vi "hReadChannels-UandP.vi"(0 "FPGA VI Reference In":refnum<k20>, 1 "SavGol side points":i32=10, 3 "Use Voltage or Power for AO?":bool, 4 "order polynomial":i32=2, 5 "Nsamples":u32=10000, 6 "error in":errorcluster, 8 "output cluster":T3, 9 "No. Of Samples to average":i32=5, 10 "variables cluster":T2, 11 "Calc Selection":u16(ring)=2 items=["0.4 ms", "0.8 ms", "1.6 ms", "3.2 ms", "6.4 ms", "12.8 ms"], 14 "skip feedback":bool) -> (2 "Fehler":bool, 13 "AdjustedArray":sgl[][](array[numeric]), 17 "loop DAQ timing":dbl, 18 "single channel voltage array":dbl[](array[numeric]), 19 "real time P_rad array":dbl[](array[numeric]), 20 "FPGA VI Reference Out":refnum<k20>, 22 "PowerArray":sgl[][](array[numeric]), 25 "RawArray":sgl[][](array[numeric]), 26 "error out":errorcluster)   [LabVIEW 2014]
doc: "startet das einlesen und führt dies bis n Samples aus\nHier mit FIFO und IRQ."
uses:
  <vilib>/Utility/error.llb/Error Cluster From Error Code.vi
  <vilib>/rvi/errors/niLvFpgaAdjustHostInterfaceError.vi
  <vilib>/RVI Host/nirviSupport.llb/nirviErrorClusterFromErrorCode.vi
  <vilib>/rvi/interface/nirviReadWriteControl/nirviReadWriteControl.xnode
  FPGA Bitfiles/W7XBolo2017_FPGATarget_fmain2014_DACRangeVoltage.lvbitx
  f_main_2014.vi
  <vilib>/rvi/interface/nirviMethod/nirviMethod.xnode
  NiFpgaLv.dll
  <vilib>/rvi/interface/nirviMethod/StockFPGA_InlinedMethodWaitForMultipleIRQ.vi
  <vilib>/FPGAPlugInAG/PCI-7813R/niLvFpga_WaitOnIrq_PCI-7813R.vi
  <vilib>/FPGAPlugInAG/PCI-7813R/niLvFpga_AcknowledgeIrq_PCI-7813R.vi
  <vilib>/FPGAPlugInAG/PCI-7813R/niLvFpga_ReadFifo_PCI-7813R.vi
  <vilib>/rvi/errors/niLvFpgaMergeErrorWithErrorCode.vi
panel:
  in  "Tab Control":T1(tab)
  out "16bit integer voltage sample":i16[](array[numeric])
  out "Timed Out":bool
  out "STOP?":bool
  out "Elements Remaining":u32
  out "single channel voltage":sgl
  out "single channel voltage * factor":dbl
  out "empty sample array":dbl[](array[numeric])
  out "Nsamples array":i64[](array[numeric])
  out "new level of override":i32=1565
  out "last U sample":sgl[](array[numeric])=[-7.323455e-08, 6.4667313e-07, 1.2200326e-06, -9.891577e-07, -1.4648394e-06, 8.4836154e-07, 0.0, -1.0253722e-06, -6.349012e-07, 2.9421412e-06, 1.8309802e-06, -1.6723759e-06, -8.0589206e-07, 1.2935698e-06, 1.2819655e-06, -1.355093e-06, -3.7858263e-07, 5.865097e-07, 5.370006e-07, -3.6600977e-07, 0.0, -4.235832e-06, 7.87382e-07, -8.300087e-07, -2.3216009e-07, 6.100163e-07, 4.6361237e-07, -4.2733737e-07, -1.1170097e-06, 4.6361237e-07, 6.4709224e-07, -9.032898e-07, 0.0, -3.600493e-07, -9.394251e-07, 7.939525e-07, 9.028241e-07, -9.2692676e-07, 6.595068e-07, -1.5255064e-06, -1.1291402e-06, 1.257381e-06, -1.1108303e-06, 1.4649238e-06, -8.564442e-08, -5.254149e-07, 5.859509e-07, -5.5879357e-10, -5.3096096e-07, 1.4771707e-06, 1.0997057e-07, -1.416197e-06, -6.2856355e-07, -8.4228816e-07, -1.6051717e-06, -8.0560335e-07, -2.3067928e-06, -1.1781231e-06, 1.4042482e-06, -1.1242553e-05, -2.111881e-06, 1.9225524e-06, -6.4575115e-06, 2.1361745e-07, 2.5024683e-06, -3.6619604e-06, -2.1238252e-06, -3.6375504e-06, -2.7460046e-06, 1.2200326e-06, 1.1045952e-06, -8.5447914e-07, -2.282681e-06, 0.0, 2.4409965e-06, 6.100163e-07, -5.0041825e-07, -1.842957e-06, -3.2471494e-06, -8.7925235e-07, 1.5277057e-05, 3.460478e-06, 2.8060748e-07, -2.3826956e-07, -2.3319571e-06, 1.3062544e-06, 5.428121e-07, 0.0, 6.6523904e-07, -1.2820121e-07, -2.563931e-06, -7.8128653e-07, -1.5884638e-07, 2.1481887e-06, 3.747493e-06, 4.270114e-07, -1.0980293e-07, -7.0789827e-07, -2.3180618e-07, 4.3368087e-19, -1.2810342e-07, 4.8801303e-07, 6.8413095e-07, 3.054738e-07, 1.830794e-07, 4.0261074e-07, -1.3440848e-07, -6.469898e-07, -8.1180593e-07, 7.629387e-07, 9.583147e-07, -1.2207033e-07, -8.54861e-07, 0.0, -2.6020852e-18, -1.7347235e-18, 2.6020852e-18, -5.2041704e-18, 0.0, -4.3368087e-18, -5.2041704e-18, 6.071532e-18, 0.0, -6.071532e-18, -5.2041704e-18, 3.469447e-18, 8.6736174e-19, 4.882812e-07]
  out "rt prad average array":dbl[][](array[numeric])=[[16187.230458648359, 1.7790693343739788e-06, 1.6846550453348635e-06, 1.590240756295748e-06, -1.4169350553503868e-06, 1.873483623413094e-06], [6006.187701750158, 1.5812885465236652e-06, 0.0, 0.0, 0.0, 1.6310928420092047e-06], [-7733.12552392997, -1.343402214503583e-06, -1.343402214503583e-06, -1.343402214503583e-06, -1.343402214503583e-06, -1.343402214503583e-06], [1286.0041024405336, 2.1500197352911071e-07, 2.1500197352911071e-07, 2.1500197352911071e-07, 2.1500197352911071e-07, 2.1500197352911071e-07], [10742.914497971773, 1.6630036445855612e-06, 1.6385408995701998e-06, 2.3844033590826234e-06, 1.565155624694354e-06, 1.687466389600928e-06]]
  out "prad av array":dbl[](array[numeric])
  out "index status":bool
  out "channel number":i64
  out "RawScal":dbl[](array[numeric])
  out "Scale(mV)":sgl[](array[numeric])
  out "SumScal":dbl[](array[numeric])
  out "Tau/dt":dbl[](array[numeric])
  out "F_ch":dbl[](array[numeric])
  out "tau_fact":dbl[](array[numeric])
  out "kbolott_and_volume":dbl[][](array[numeric])=[[1e-05, 1e-05], [9.8364458e-05, 1.8160732], [0.00029863964, 770.25441], [0.00053910452, 1653.5432], [0.00071569496, 2554.7619], [0.00083348142, 3356.1809], [0.00092645429, 4021.9678], [0.00099241932, 4570.4466], [0.0010332482, 4989.6792], [0.0010552469, 5170.4882], [0.0010669981, 5192.5645], [0.001071534, 5152.6222], [0.0010766644, 5109.6704], [0.0010841289, 5094.9972], [0.0010884845, 5078.237], [0.0010888843, 5058.9416], [0.0010882289, 5056.581], [0.0010872861, 5078.1684], [0.0010832221, 5096.5196], [0.0010760805, 5113.7904], [0.0010685167, 5141.4566], [0.0010644166, 5189.7831], [0.0010539441, 5182.7365], [0.0010337779, 5034.6928], [0.00098716411, 4625.8518], [0.00091599422, 4090.3707], [0.00082376071, 3438.9665], [0.00070194108, 2659.5109], [0.00051785958, 1753.3355], [0.00030745544, 937.82125], [0.00014081292, 59.55205], [1e-05, 1e-05], [0.0, 0.0], [0.0, 0.0], [0.0, 0.0], [0.0, 0.0], [0.0, 0.0], [0.0, 0.0], [0.0, 0.0], [0.0, 0.0], [0.0, 0.0], [0.0, 0.0], [0.0, 0.0], [0.0, 0.0], [0.0, 0.0], [0.0, 0.0], [0.0, 0.0], [0.0, 0.0], [0.0019134875, 3474.3085], [0.0020594744, 3690.1455], [0.002175929, 3861.3028], [0.0022530617, 3956.5918], [0.0023492529, 4057.9903], [0.0024581424, 4205.0841], [0.0025383764, 4324.9746], [0.0025876415, 4417.9525], [0.0026676725, 4566.0612], [0.0027635964, 4770.6296], [0.0028188521, 4914.295], [0.0028263806, 4970.0105], [0.0028491244, 5014.7926], [0.0028762033, 5060.279], [0.0028430703, 4969.1072], [0.0027058578, 4592.2853], [0.0019047772, 4936.5706], [0.0023594746, 6388.5028], [0.0025094117, 6336.5413], [0.002569351, 6048.9284], [0.0026367277, 5794.3031], [0.002714522, 5668.1597], [0.0027530637, 5505.217], [0.0027520905, 5312.6378], [0.0027781484, 5183.8321], [0.0028283925, 5165.5044], [0.0028425709, 5118.655], [0.00281436, 5016.5122], [0.0027996491, 4909.784], [0.0027993913, 4845.125], [0.0027603692, 4728.4661], [0.0026886073, 4585.7454], [0.0026437627, 4495.4419], [0.0026242501, 4486.7206], [0.0025685332, 4434.986], [0.0024747416, 4324.8822], [0.0023915919, 4209.8149], [0.002319616, 4111.844], [0.0022042921, 3923.4955], [0.0020485146, 3644.5259], [0.0024033884, 3597.1969], [0.002066694, 2566.1598], [0.0017718795, 1878.4004], [0.0015136288, 1414.3006], [0.0013043692, 1094.5581], [0.0011378765, 882.65731], [0.00097324167, 712.97006], [0.00080739571, 571.52867], [0.0, 0.0], [0.0, 0.0], [0.0, 0.0], [0.0, 0.0], [0.0, 0.0], [0.0, 0.0], [0.0, 0.0], [0.0, 0.0], [0.0, 0.0], [0.0, 0.0], [0.0, 0.0], [0.0, 0.0], [0.0, 0.0], [0.0, 0.0], [0.0, 0.0], [0.0, 0.0], [0.0, 0.0], [0.0, 0.0], [0.0, 0.0], [0.0, 0.0], [0.0, 0.0], [0.0, 0.0], [0.0, 0.0], [0.0, 0.0], [0.0, 0.0], [0.0, 0.0], [0.0, 0.0], [0.0, 0.0], [0.0, 0.0], [0.0, 0.0], [0.0, 0.0], [0.0, 0.0]]
  out "single channel number":i64=70
  out "channelNumber":i32=5
  out "channelSelection":i64[][](array[numeric])=[[65], [73], [78], [86], [61]]
  out "tau_M":dbl[](array[numeric])
  out "Offsets":dbl[](array[numeric])
  out "SampleTime":sgl=0.0032
  out "voltage factor":dbl=17500.0
  out "Scale(mV) transf.":sgl[](array[numeric])
  out "V_cam":dbl=25266.247799999997
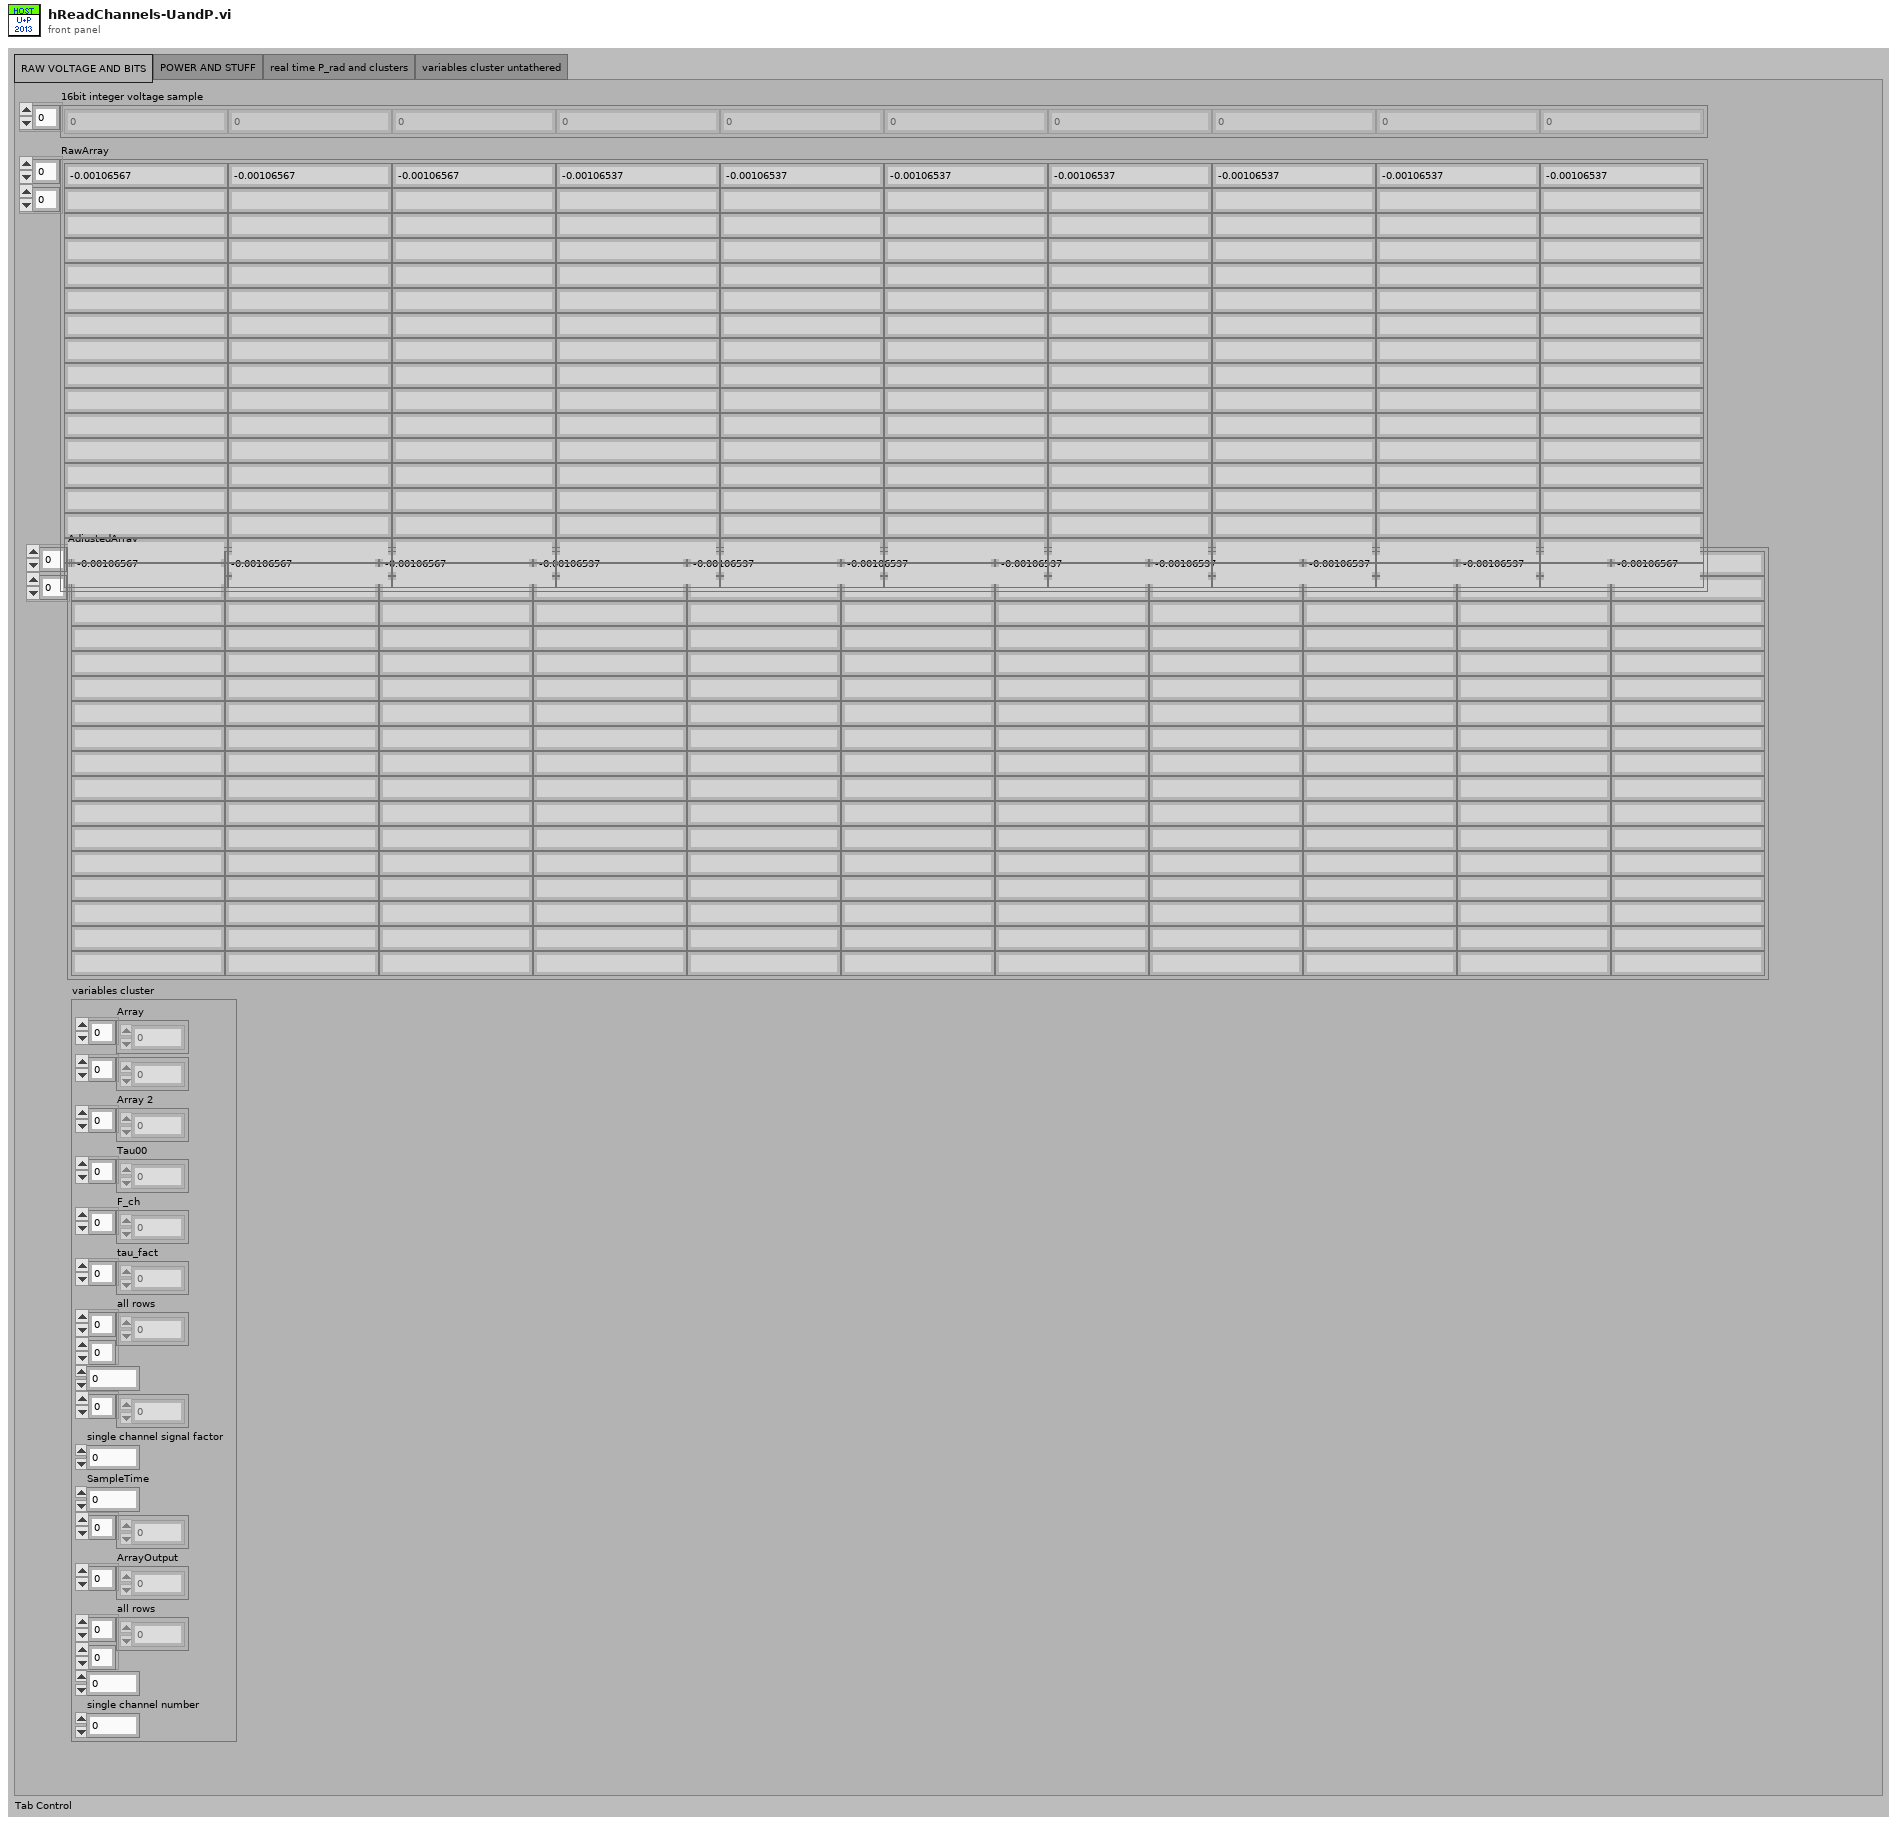
[diagram p1: front panel]
types:
  T1 = enum32{"RAW VOLTAGE AND BITS", "POWER AND STUFF", "real time P_rad and clusters", "variables cluster untathered"}
  T2 = cluster{"Array":dbl[], sgl[], "Array 2":dbl[], "Tau00":dbl[], "F_ch":dbl[], "tau_fact":dbl[], "all rows":dbl[][], dbl, sgl[], "single channel signal factor":dbl, "SampleTime":sgl, dbl[], "ArrayOutput":dbl[], "all rows":i64[][], i32, "single channel number":i64}
  T3 = cluster{"real time P_rad":refnum<vi>, "real time P_rad array":refnum<vi>, "single channel voltage":refnum<vi>, "single channel voltage array":refnum<vi>}
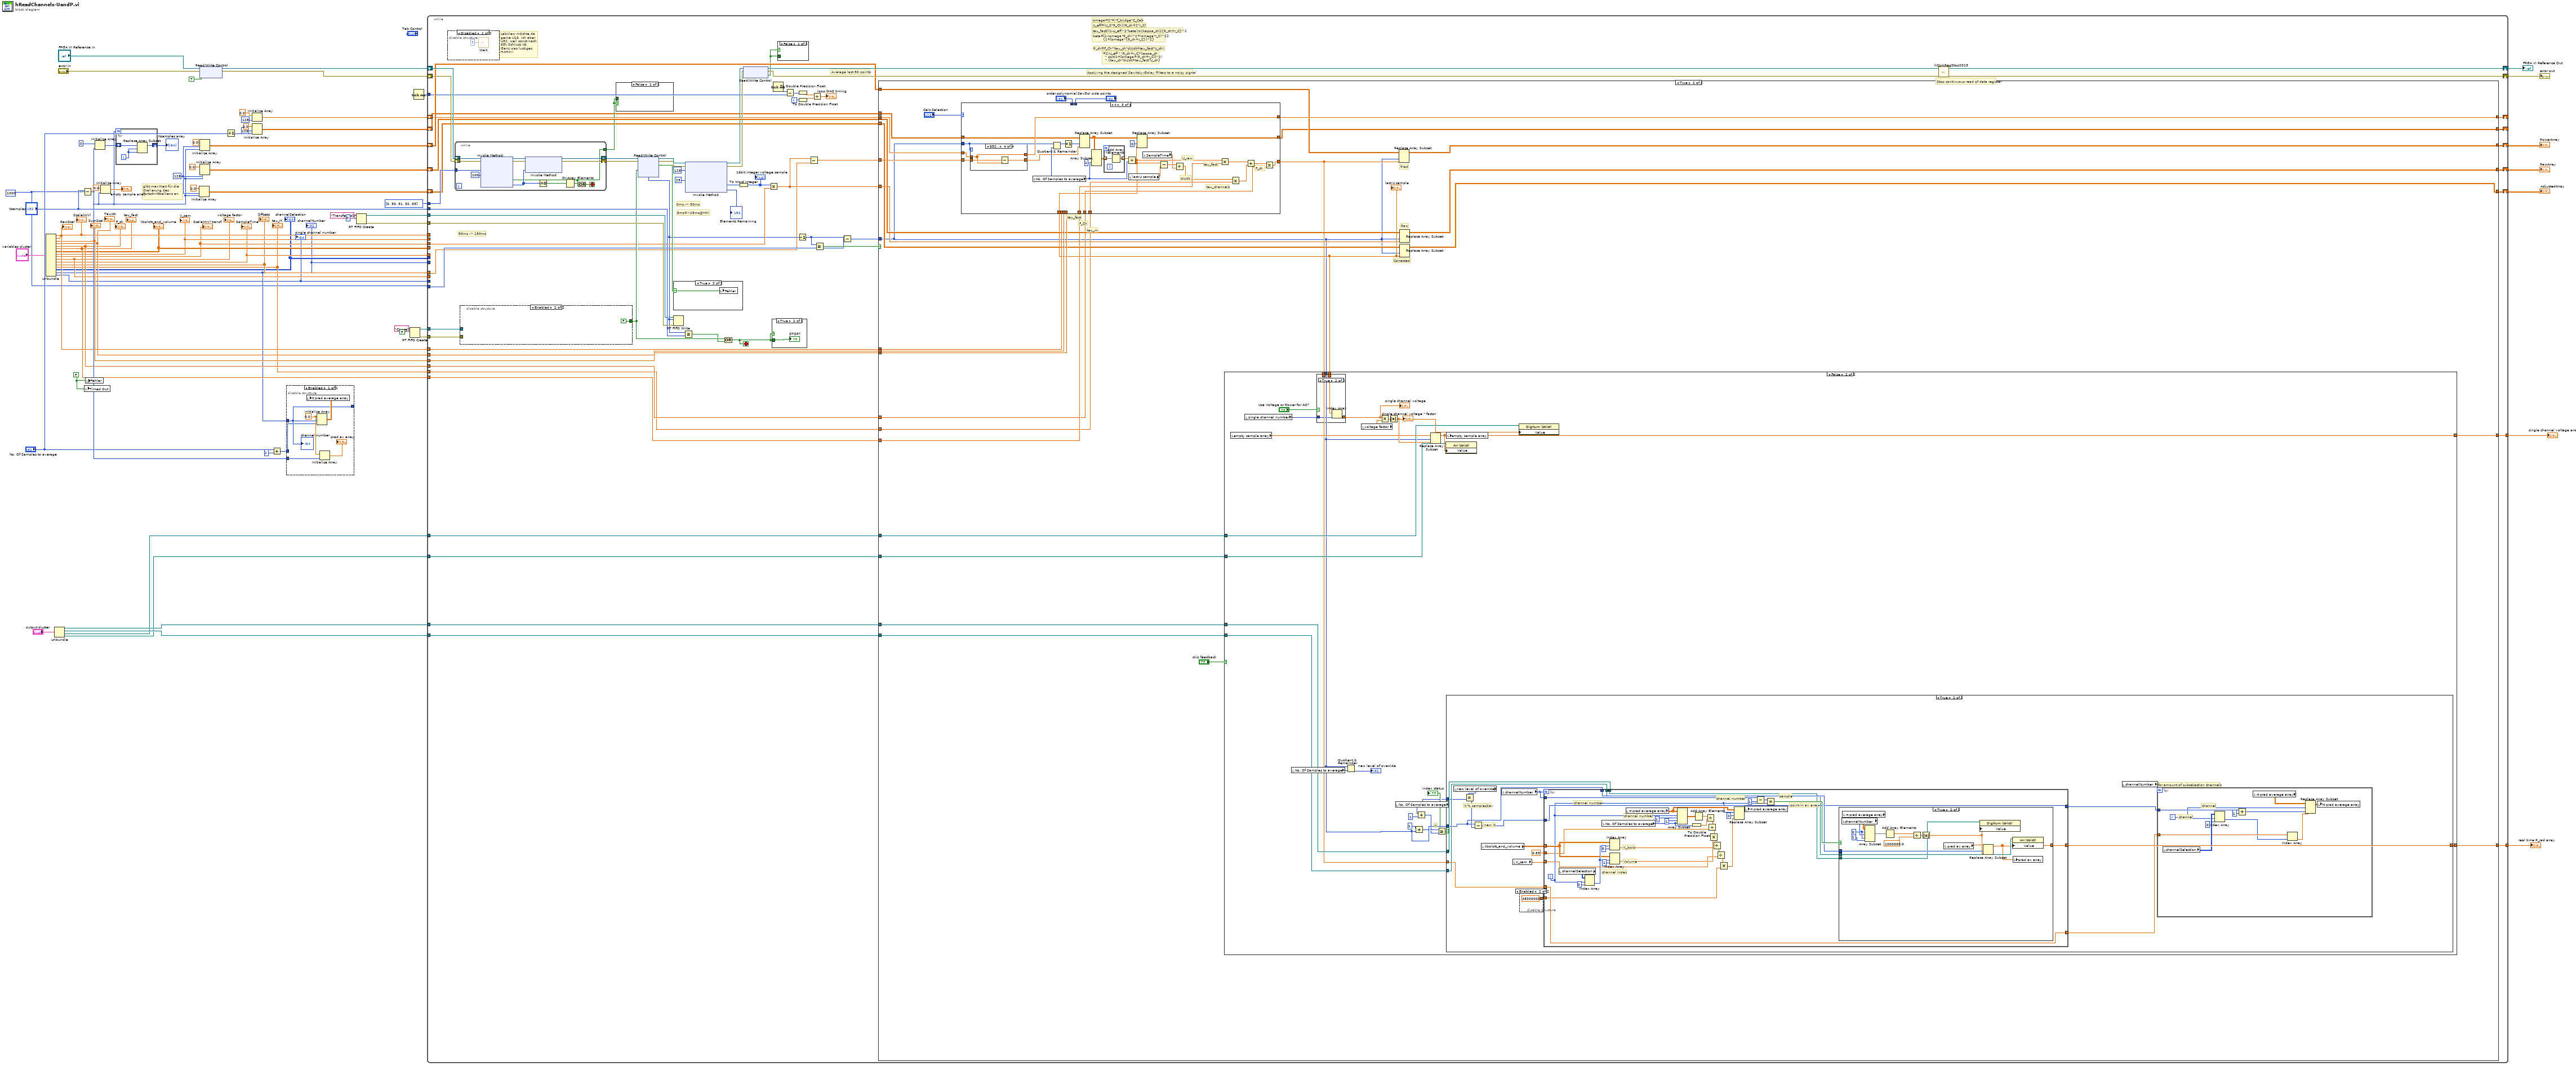
[diagram p0: block diagram]
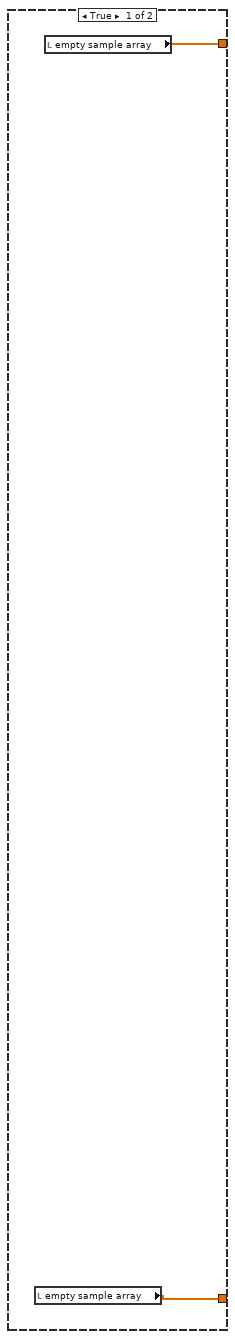
[diagram p3: hidden frame]
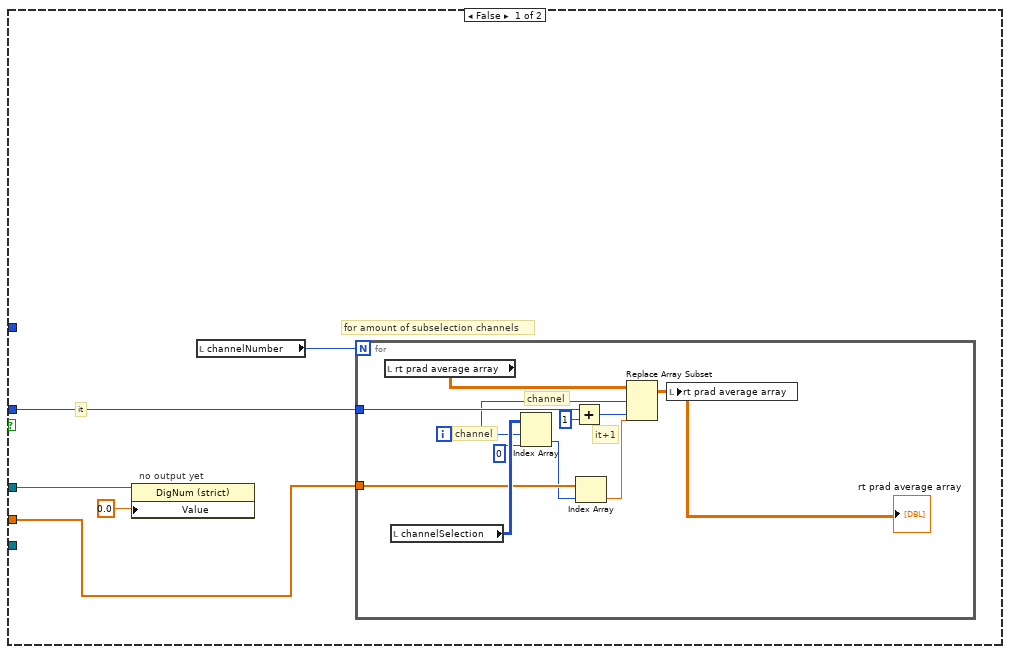
[diagram p4: hidden frame]
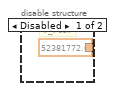
[diagram p5: hidden frame]
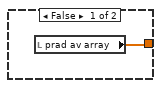
[diagram p6: hidden frame]
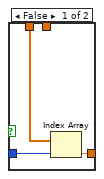
[diagram p7: hidden frame]
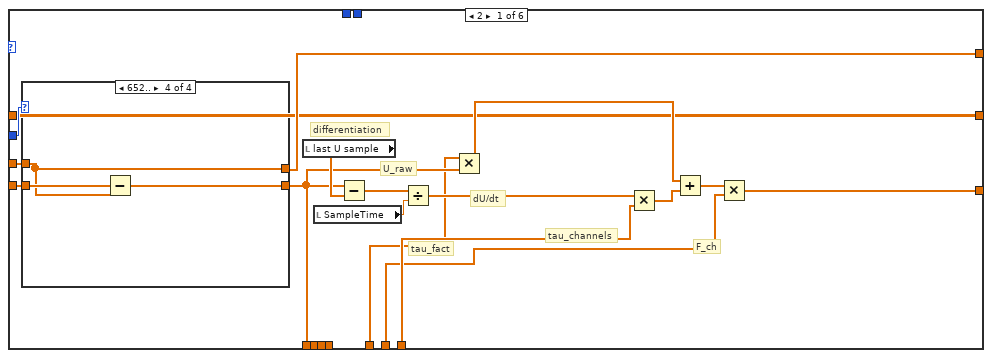
[diagram p8: hidden frame]
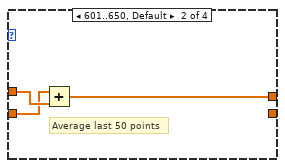
[diagram p10: hidden frame]
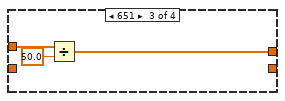
[diagram p11: hidden frame]
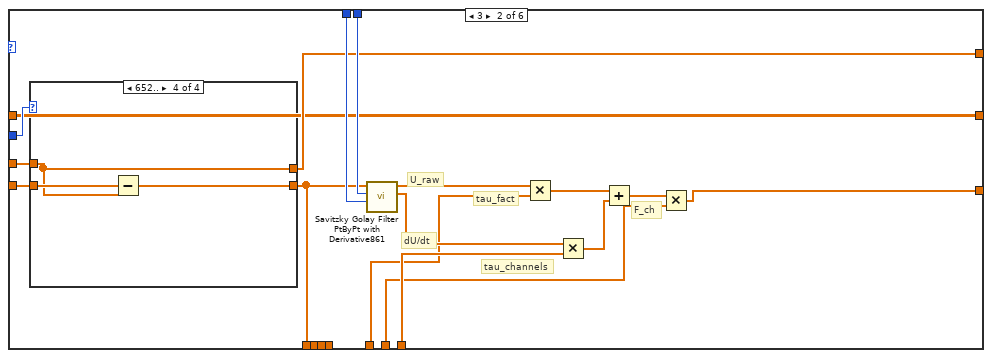
[diagram p12: hidden frame]
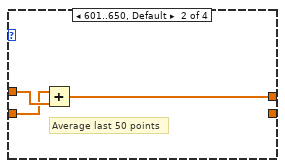
[diagram p14: hidden frame]
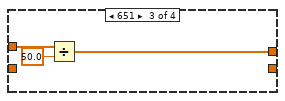
[diagram p15: hidden frame]
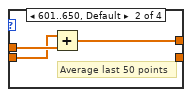
[diagram p17: hidden frame]
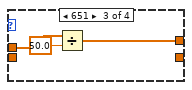
[diagram p18: hidden frame]
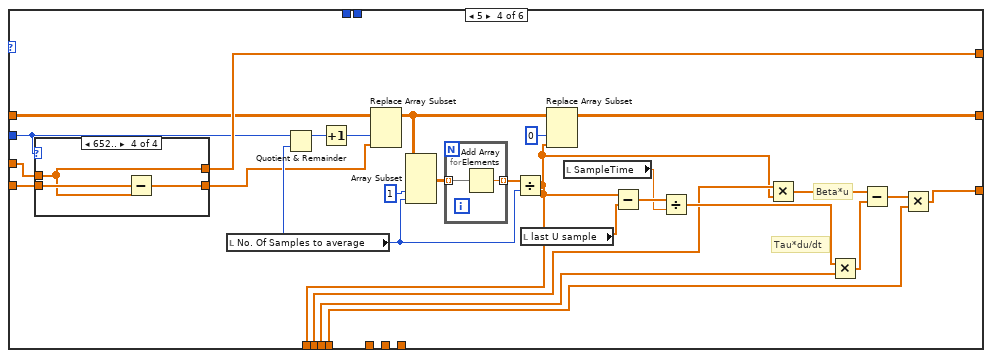
[diagram p19: hidden frame]
diagram:
  w17 = u32 1000 ("samples to exclude")
  w41 = FALSE
  w29 = 128 ("dimension size")
  # "Stop continuous read of data register"
  # "gibt maxWert für die Skalierung des Fortschrittbalkens an"
  n1 = Unbundle("variables cluster") -> ("Array"=w16:dbl[], w15:sgl[], "Array 2"=w14:dbl[], "Tau00"=w13:dbl[], "F_ch"=w12:dbl[], "tau_fact"=w11:dbl[], "all rows"=w10:dbl[][], w9:dbl, w8:sgl[], "single channel signal factor"=w7:dbl, "SampleTime"=w6:sgl, w5:dbl[], "ArrayOutput"=w4:dbl[], "all rows"=w3:i64[][], w2:i32, "single channel number"=w1:i64)
  "RawScal" <- w16
  "Scale(mV)" <- w15
  "SumScal" <- w14
  "Tau/dt" <- w13
  "F_ch" <- w12
  "tau_fact" <- w11
  "kbolott_and_volume" <- w10
  "V_cam" <- w9
  "Scale(mV) transf." <- w8
  "voltage factor" <- w7
  "SampleTime" <- w6
  "Offsets" <- w5
  "tau_M" <- w4
  "channelSelection" <- w3
  "channelNumber" <- w2
  "single channel number" <- w1
  n2 = Unbundle("output cluster") -> ("real time P_rad"=w39:refnum<vi>, "real time P_rad array"=w38:refnum<vi>, "single channel voltage"=w34:refnum<vi>, "single channel voltage array"=w33:refnum<vi>)
  n3 = Subtract(x="Nsamples", y=w17) -> (x-y=w28:u32)
  n4 = local write "Timed Out"(w41) -> ()
  n5 = local write "Fehler"(w41) -> ()
  n6 = Initialize Array(i64 0 ("element"), w28) -> (w43:i64[])
  n7 = Initialize Array(0.0 ("element"), w28) -> (→"empty sample array":dbl[])
  n8 = for {
    N: w28 -> [_]
    shift-right: [w73] -> w42
    shift-left: w43 -> [w75]
    i -> [w74]
    n9 = Replace Array Subset(array=w75, new element=w74, index=w74) -> (w73:i64[])
  }
  "Nsamples array" <- w42
  n10 = Initialize Array(sgl 0.0 ("element"), w29, w28) -> (w27:sgl[][])
  n11 = xnode "Read/Write Control"("FPGA VI Reference In"="FPGA VI Reference In", "error in"="error in", "ADCRead"=TRUE) -> ("FPGA VI Reference Out"=w54:refnum<k20>, "error out"=w53:errorcluster)
  n12 = Initialize Array(sgl 0.0 ("i"), w29, w28) -> (w63:sgl[][])
  n13 = Initialize Array(sgl 0.0, w29, w28) -> (w72:sgl[][])
  n14 = Increment(x="No. Of Samples to average") -> (x+1=w22:i32)
  n15 = Initialize Array(sgl 0.0 ("element"), 128 ("dimension size")) -> (w49:sgl[])
  n16 = Initialize Array(0.0 ("element"), 128 ("dimension size"), w22) -> (w20:dbl[][])
  n17 = Add(x="No. Of Samples to average", y=1) -> (x+y=w36:i32)
  n18 = disable-structure shown="Enabled" {
    disable-tunnel: w2 -> [w80]
    disable-tunnel: [w80] -> _
    disable-tunnel: w36 -> [w76]
    disable-tunnel: w28 -> [w77]
    frame Enabled {
      w79 = 0.0 ("element")
      n19 = Initialize Array(w79, w80, w76) -> (w81:dbl[][])
      n20 = local write "rt prad average array"(w81) -> ()
      n21 = Initialize Array(w79, w77) -> (→"prad av array":dbl[])
      "channel number" <- w80
    }
  }
  n22 = RT FIFO Create(0:"Transferred1" ("name (unnamed)"), 1:u32 0) -> (8:w69:refnum<k33>, 11:w68:errorcluster)  [unwired: 2 in, 5 out]
  n23 = RT FIFO Create(0:"Cancel" ("name (unnamed)"), 1:FALSE) -> (8:w66:refnum<k33>, 11:w65:errorcluster)  [unwired: 2 in, 5 out]
  n24 = Tick Count (ms)() -> (millisecond timer value=w19:u32)
  n25 = while {
    tunnel: "Nsamples" -> [w141]
    shift-right: [w109] -> w25
    shift-left: w72 -> [w130]
    shift-right: [w142] -> w62
    shift-left: w54 -> [w145]
    shift-right: [w143] -> w61
    shift-left: w53 -> [w144]
    tunnel: w69 -> [w140]
    tunnel: w68 -> [w139]
    tunnel: w66 -> [w137]
    tunnel: w65 -> [w136]
    shift-right: [w134] -> w57
    shift-left: w63 -> [w135]
    tunnel: w8 -> [w129]
    tunnel: w13 -> [w126]
    tunnel: w14 -> [w128]
    tunnel: w16 -> [w127]
    shift-right: [w119] -> _
    shift-left: w49 -> [w96]
    tunnel: i32[] [0, 30, 31, 32, 33] -> [w114]
    tunnel: w33 -> [w111]
    tunnel: w34 -> [w110]
    tunnel: w1 -> [_]
    tunnel: w7 -> [_]
    tunnel: w5 -> [w92]
    tunnel: w17 -> [w93]
    tunnel: w39 -> [w106]
    tunnel: w38 -> [w102]
    tunnel: w12 -> [w105]
    tunnel: w11 -> [w91]
    tunnel: w15 -> [_]
    tunnel: w10 -> [_]
    tunnel: w6 -> [_]
    tunnel: w4 -> [w104]
    tunnel: w3 -> [_]
    tunnel: w2 -> [_]
    tunnel: w9 -> [_]
    tunnel: [w101] -> w32
    tunnel: [w100] -> w31
    shift-right: [w98] -> w26
    shift-left: w27 -> [w99]
    shift-right: [w89] -> _
    shift-left: w20 -> [w90]
    tunnel: w19 -> [w87]
    i -> [w85]
    stop <- w115 stop-if-true
    # "beta=[1-(omega*R_ch)^2+(omega*r_C)^2]/\n         {1+[omega*{R_ch+r_C}]^2}"
    # "tau_fact[((1-U_eff^2*beta)/4)/kappa_ch]/{R_ch+r_C}^2"
    # "U_eff=(U_0*R_Ch)/(R_ch+2*r_C)"
    # "omega=2*Pi*f_bridge*C_Cab"
    # "=2/U_eff * (R_ch+r_C)*kappa_ch\n  * sqrt(1+[omega+(R_ch+r_C)]^2)\n  * {tau_ch*dU/dt+tau_fact*U_ch}"
    # "P_ch=F_Ch*(tau_ch*dU/dt+tau_fact*U_ch)"
    # "Average last 50 points"
    # "Applying the designed Savitzky-Golay Filters to a noisy signal"
    # "LabView möchte da gerne U16, ich aber U32, weil sonst nach 65k Schluss ist. \nGanz was lustiges, HAHA!!"
    # "5ms=>25ms@MM"
    # "0ms -> 50ms"
    # "50ms -> 150ms"
    n26 = disable-structure shown="Disabled" {
      frame Disabled {
        n27 = call "Wait"("Count(uSec)"=u32 5) -> ()  [unwired: 1 out]
      }
      frame Enabled {
      }
    }
    n28 = while {
      tunnel: [w505] -> w118
      shift-right: [w507] -> w112
      shift-left: w145 -> [w514]
      shift-right: [w506] -> w113
      shift-left: w144 -> [w513]
      tunnel: w114 -> [w511]
      stop <- w504 stop-if-true
      n29 = xnode "Invoke Method"("FPGA VI Reference In"=w514, "error in"=w513, "IRQ Number(s)"=w511, "Timeout (ms)"=100) -> ("FPGA VI Reference Out"=w508:refnum<k20>, "error out"=w509:errorcluster, "Timed Out"=w505:bool, "IRQ(s) Asserted"=w510:i32[])
      n30 = xnode "Invoke Method"("FPGA VI Reference In"=w508, "error in"=w509, "IRQ Number(s)"=w510) -> ("FPGA VI Reference Out"=w507:refnum<k20>, "error out"=w506:errorcluster)
      n31 = Equal To 0?(x=w510) -> (x = 0?=w503:bool[])
      n32 = Or Array Elements(Boolean array=w503) -> (logical OR=w502:bool)
      n33 = Or(x=w502, y=w505) -> (x .or. y?=w504:bool)
    }
    n34 = disable-structure shown="Enabled" {
      disable-tunnel: [w520 FALSE] -> w138
      disable-tunnel: w137 -> [w519 _]
      disable-tunnel: w136 -> [w518 _]
      frame Disabled {
        # "Da es passieren kann, dass der letzte IRQ verschluckt wird, sichert dies der Timeoutwert von 50ms ab."
        n35 = RT FIFO Read(0:w519, 1:FALSE ("element"), 3:w518) -> (9:w520:bool)  [unwired: 5 out]
      }
      frame Enabled {
      }
    }
    n36 = case shown="False" w118 {
      tunnel: w118 -> [_ w522]
      frame False {
      }
      frame True {
        "Timed Out" <- w522
      }
    }
    n37 = xnode "Read/Write Control"("FPGA VI Reference In"=w112, "error in"=w113, "cancel"=w138) -> ("FPGA VI Reference Out"=w132:refnum<k20>, "error out"=w131:errorcluster, "Timeout"=w133:bool, "ScanID"=w97:u32)
    n38 = case shown="True" w133 {
      selector: w133 -> [_ w524]
      frame False {
      }
      frame True {
        n39 = local write "Fehler"(w524) -> ()
      }
    }
    n40 = RT FIFO Write(0:w140, 1:w97, 3:w139) -> ()  [unwired: 1 in, 5 out]
    n41 = Greater Or Equal?(x=w97, y=w141) -> (x >= y?=w146:bool)
    n42 = xnode ("Invoke Method")("FPGA VI Reference In"=w132, "error in"=w131, "Number of Elements"=u32 128, "Timeout (ms)"=25 ("Timeout")) -> ("FPGA VI Reference Out"=w121:refnum<k20>, "error out"=w120:errorcluster, "Data"=w123:u32[], "Elements Remaining"=→"Elements Remaining":u32)
    n43 = Compound Arithmetic op=OR(w138, w146) -> (w115:bool)
    n44 = To Word Integer(number=w123) -> (16bit integer=w122:i16[])
    "16bit integer voltage sample" <- w122
    n45 = xnode "Read/Write Control"("FPGA VI Reference In"=w121, "error in"=w120) -> ("FPGA VI Reference Out"=w142:refnum<k20>, "error out"=w143:errorcluster, "Fifo-Fehler"=w116:bool)
    n46 = Multiply(x=w122, y=w129) -> (x*y=w95:sgl[])
    n47 = case shown="True" w115 {
      tunnel: w115 -> [_ w515]
      frame False {
      }
      frame True {
        "STOP?" <- w515
      }
    }
    n48 = Tick Count (ms)() -> (millisecond timer value=w88:u32)
    n49 = case shown="False" w116 {
      tunnel: w116 -> [_ w516]
      frame False {
      }
      frame True {
        "Fehler" <- w516
      }
    }
    n50 = Subtract(x=w88, y=w87) -> (x-y=w86:u32)
    n51 = Decrement(x=w97) -> (x-1=w107:u32)
    n52 = To Double Precision Float(number=w86) -> (double precision float=w84:dbl)
    n53 = To Double Precision Float(number=w85) -> (double precision float=w83:dbl)
    n54 = Subtract(x=w95, y=w92) -> (x-y=w94:dbl[])
    n55 = Divide(x=w84, y=w83) -> (x/y=→"loop DAQ timing":dbl)
    n56 = Greater Or Equal?(x=w107, y=w93) -> (x >= y?=w108:bool)
    n57 = Subtract(x=w107, y=w93) -> (x-y=w103:u32)
    n58 = case shown="True" w108 {
      tunnel: w135 -> [w150 w175]
      tunnel: [w150 w176] -> w134
      tunnel: w130 -> [w149 w174]
      tunnel: w128 -> [_ w182]
      tunnel: w127 -> [_ w181]
      tunnel: w126 -> [_ w180]
      tunnel: [w151 w179] -> w119
      tunnel: w96 -> [w151 w166]
      tunnel: w95 -> [_ w165]
      tunnel: w111 -> [_ w178]
      tunnel: w110 -> [_ w177]
      tunnel: [w149 w173] -> w109
      tunnel: w103 -> [_ w153]
      tunnel: w106 -> [_ w172]
      tunnel: w102 -> [_ w171]
      tunnel: w105 -> [_ w159]
      tunnel: w91 -> [_ w160]
      tunnel: w104 -> [_ w158]
      tunnel: [_ w170] -> w101
      tunnel: [_ w169] -> w100
      tunnel: w99 -> [w148 w168]
      tunnel: [w148 w167] -> w98
      tunnel: w94 -> [_ w164]
      tunnel: w90 -> [w147 w155]
      tunnel: [w147 w154] -> w89
      frame False {
      }
      frame True {
        # "Prad"
        # "tau_fact"
        # "tau_m"
        # "F_Ch"
        # "Corrected"
        # "Raw"
        n59 = case shown="4" "Calc Selection" {
          tunnel: w182 -> [_ _ _ w407 w464 w491]
          tunnel: w181 -> [_ _ _ w410 w463 w490]
          tunnel: w180 -> [_ _ _ w408 w462 w489]
          tunnel: [w320 w343 w384 w430 w461 w488] -> w179
          tunnel: w166 -> [w322 w351 w390 w432 w460 w487]
          tunnel: w153 -> [w314 w341 w375 w421 w459 w486]
          tunnel: [w315 w344 w385 w406 w458 w481] -> w156
          tunnel: "SavGol side points" -> [_ w348 _ _ w457 w485]
          tunnel: "order polynomial" -> [_ w349 _ _ w456 w484]
          tunnel: w164 -> [w321 w350 w389 w431 w455 w483]
          tunnel: [w318 w342 w370 w409 w454 w482] -> w163
          tunnel: w160 -> [w317 w346 w387 _ _ _]
          tunnel: w159 -> [w316 w345 w386 _ _ _]
          tunnel: w158 -> [w319 w347 w388 _ _ _]
          tunnel: w155 -> [w313 w340 w373 w419 w445 w475]
          tunnel: [w313 w340 w372 w418 w445 w475] -> w154
          frame 2 {
            # "differentiation"
            # "tau_channels"
            # "F_ch"
            # "tau_fact"
            # "U_raw"
            # "dU/dt"
            n60 = case shown="652.." w314 {
              tunnel: w321 -> [_ w331 _ w339]
              tunnel: [w330 w333 w334 w338] -> w320
              tunnel: w322 -> [w330 w332 w336 w338]
              tunnel: [_ _ _ w337] -> w318
              frame 0..600 {
              }
              frame 601..650, Default {
                # "Average last 50 points"
                n61 = Add(x=w331, y=w332) -> (x+y=w333:dbl[])
              }
              frame 651 {
                n62 = Divide(x=w336, y=sgl 50.0) -> (x/y=w334:dbl[])
              }
              frame 652.. {
                n63 = Subtract(x=w339, y=w338) -> (x-y=w337:dbl[])
              }
            }
            n64 = local read "last U sample"() -> (w324:sgl[])
            n65 = local read "SampleTime"() -> (w325:sgl)
            n66 = Subtract(x=w318, y=w324) -> (x-y=w323:dbl[])
            n67 = Divide(x=w323, y=w325) -> (x/y=w326:dbl[])
            n68 = Multiply(x=w317, y=w318) -> (x*y=w329:dbl[])
            n69 = Multiply(x=w326, y=w319) -> (x*y=w327:dbl[])
            n70 = Add(x=w329, y=w327) -> (x+y=w328:dbl[])
            n71 = Multiply(x=w328, y=w316) -> (x*y=w315:dbl[])
          }
          frame 3 {
            # "tau_channels"
            # "F_ch"
            # "tau_fact"
            # "U_raw"
            # "dU/dt"
            n72 = case shown="652.." w341 {
              tunnel: w350 -> [_ w358 _ w366]
              tunnel: [w357 w360 w361 w365] -> w343
              tunnel: w351 -> [w357 w359 w363 w365]
              tunnel: [_ _ _ w364] -> w342
              frame 0..600 {
              }
              frame 601..650, Default {
                # "Average last 50 points"
                n73 = Add(x=w358, y=w359) -> (x+y=w360:dbl[])
              }
              frame 651 {
                n74 = Divide(x=w363, y=sgl 50.0) -> (x/y=w361:dbl[])
              }
              frame 652.. {
                n75 = Subtract(x=w366, y=w365) -> (x-y=w364:dbl[])
              }
            }
            n76 = call "Savitzky Golay Filter PtByPt with Derivative861.vi"("order polynomial"=w349, "side points"=w348, "x"=w342) -> ("Filtered Derivative"=w353:dbl[], "Filtered x"=w352:dbl[])  [unwired: 1 in, 6 out]
            n77 = Multiply(x=w352, y=w346) -> (x*y=w356:dbl[])
            n78 = Multiply(x=w353, y=w347) -> (x*y=w354:dbl[])
            n79 = Add(x=w356, y=w354) -> (x+y=w355:dbl[])
            n80 = Multiply(x=w355, y=w345) -> (x*y=w344:dbl[])
          }
          frame 4 {
            # "tau_channels"
            # "F_ch"
            # "tau_fact"
            # "U_raw"
            # "dU/dt"
            n81 = case shown="652.." w375 {
              tunnel: w389 -> [_ w397 _ w405]
              tunnel: [w396 w399 w400 w404] -> w384
              tunnel: w390 -> [w396 w398 w402 w404]
              tunnel: [_ _ _ w403] -> w374
              frame 0..600 {
              }
              frame 601..650, Default {
                # "Average last 50 points"
                n82 = Add(x=w397, y=w398) -> (x+y=w399:dbl[])
              }
              frame 651 {
                n83 = Divide(x=w402, y=sgl 50.0) -> (x/y=w400:dbl[])
              }
              frame 652.. {
                n84 = Subtract(x=w405, y=w404) -> (x-y=w403:dbl[])
              }
            }
            n85 = local read "No. Of Samples to average"() -> (w383:i32)
            n86 = Quotient & Remainder(x=w375, y=w383) -> (x-y*floor(x/y)=w376:u32)  [unwired: 1 out]
            n87 = Increment(x=w376) -> (x+1=w377:u32)
            n88 = Replace Array Subset(array=w373, new element=w374, index (col)=w377) -> (w381:dbl[][])  [unwired: 1 in]
            n89 = Array Subset(array=w381, index (col)=1 ("index"), length (col)=w383) -> (w380:dbl[][])  [unwired: 2 in]
            n90 = for {
              tunnel: w380 -> [w395] mode=indexing
              tunnel: [w394] -> w379 mode=indexing
              n91 = Add Array Elements(numeric array=w395) -> (sum=w394:dbl)
            }
            n92 = Divide(x=w379, y=w383) -> (x/y=w370:dbl[])
            n93 = local read "last U sample"() -> (w369:sgl[])
            n94 = Replace Array Subset(array=w381, new element=w370, index (col)=0 ("disabled index (col)")) -> (w372:dbl[][])  [unwired: 1 in]
            n95 = local read "SampleTime"() -> (w368:sgl)
            n96 = Subtract(x=w370, y=w369) -> (x-y=w371:dbl[])
            n97 = Divide(x=w371, y=w368) -> (x/y=w367:dbl[])
            n98 = Multiply(x=w370, y=w387) -> (x*y=w393:dbl[])
            n99 = Multiply(x=w367, y=w388) -> (x*y=w391:dbl[])
            n100 = Add(x=w393, y=w391) -> (x+y=w392:dbl[])
            n101 = Multiply(x=w392, y=w386) -> (x*y=w385:dbl[])
          }
          frame 5 {
            # "Beta*u"
            # "Tau*du/dt"
            n102 = case shown="652.." w421 {
              tunnel: w431 -> [_ w436 _ w444]
              tunnel: [w435 w438 w439 w443] -> w430
              tunnel: w432 -> [w435 w437 w441 w443]
              tunnel: [_ _ _ w442] -> w420
              frame 0..600 {
              }
              frame 601..650, Default {
                # "Average last 50 points"
                n103 = Add(x=w436, y=w437) -> (x+y=w438:dbl[])
              }
              frame 651 {
                n104 = Divide(x=w441, y=sgl 50.0) -> (x/y=w439:dbl[])
              }
              frame 652.. {
                n105 = Subtract(x=w444, y=w443) -> (x-y=w442:dbl[])
              }
            }
            n106 = local read "No. Of Samples to average"() -> (w429:i32)
            n107 = Quotient & Remainder(x=w421, y=w429) -> (x-y*floor(x/y)=w422:u32)  [unwired: 1 out]
            n108 = Increment(x=w422) -> (x+1=w423:u32)
            n109 = Replace Array Subset(array=w419, new element=w420, index (col)=w423) -> (w427:dbl[][])  [unwired: 1 in]
            n110 = Array Subset(array=w427, index (col)=1 ("index"), length (col)=w429) -> (w426:dbl[][])  [unwired: 2 in]
            n111 = for {
              tunnel: w426 -> [w434] mode=indexing
              tunnel: [w433] -> w425 mode=indexing
              n112 = Add Array Elements(numeric array=w434) -> (sum=w433:dbl)
            }
            n113 = Divide(x=w425, y=w429) -> (x/y=w409:dbl[])
            n114 = local read "last U sample"() -> (w416:sgl[])
            n115 = Replace Array Subset(array=w427, new element=w409, index (col)=0 ("disabled index (col)")) -> (w418:dbl[][])  [unwired: 1 in]
            n116 = local read "SampleTime"() -> (w415:sgl)
            n117 = Subtract(x=w409, y=w416) -> (x-y=w417:dbl[])
            n118 = Divide(x=w417, y=w415) -> (x/y=w411:dbl[])
            n119 = Multiply(x=w410, y=w409) -> (x*y=w414:dbl[])
            n120 = Multiply(x=w411, y=w408) -> (x*y=w412:dbl[])
            n121 = Subtract(x=w414, y=w412) -> (x-y=w413:dbl[])
            n122 = Multiply(x=w413, y=w407) -> (x*y=w406:dbl[])
          }
          frame 0 {
            # "Beta*u"
            # "Tau*du/dt"
            n123 = case shown="652.." w459 {
              tunnel: w455 -> [_ w466 _ w474]
              tunnel: [w465 w468 w469 w473] -> w461
              tunnel: w460 -> [w465 w467 w471 w473]
              tunnel: [_ _ _ w472] -> w454
              frame 0..600 {
              }
              frame 601..650, Default {
                # "Average last 50 points"
                n124 = Add(x=w466, y=w467) -> (x+y=w468:dbl[])
              }
              frame 651 {
                n125 = Divide(x=w471, y=sgl 50.0) -> (x/y=w469:dbl[])
              }
              frame 652.. {
                n126 = Subtract(x=w474, y=w473) -> (x-y=w472:dbl[])
              }
            }
            n127 = call "Savitzky Golay Filter PtByPt with Derivative861.vi"("order polynomial"=w456, "side points"=w457, "x"=w454) -> ("Filtered x"=w446:dbl[])  [unwired: 1 in, 7 out]
            n128 = local read "last U sample"() -> (w448:sgl[])
            n129 = Subtract(x=w446, y=w448) -> (x-y=w449:dbl[])
            n130 = local read "SampleTime"() -> (w447:sgl)
            n131 = Divide(x=w449, y=w447) -> (x/y=w451:dbl[])
            n132 = Multiply(x=w463, y=w446) -> (x*y=w453:dbl[])
            n133 = Multiply(x=w451, y=w462) -> (x*y=w450:dbl[])
            n134 = Subtract(x=w453, y=w450) -> (x-y=w452:dbl[])
            n135 = Multiply(x=w452, y=w464) -> (x*y=w458:dbl[])
          }
          frame 1, Default {
            # "Beta*u"
            # "Tau*du/dt"
            n136 = case shown="652.." w486 {
              tunnel: w483 -> [_ w493 _ w501]
              tunnel: [w492 w495 w496 w500] -> w488
              tunnel: w487 -> [w492 w494 w498 w500]
              tunnel: [_ _ _ w499] -> w482
              frame 0..600 {
              }
              frame 601..650, Default {
                # "Average last 50 points"
                n137 = Add(x=w493, y=w494) -> (x+y=w495:dbl[])
              }
              frame 651 {
                n138 = Divide(x=w498, y=sgl 50.0) -> (x/y=w496:dbl[])
              }
              frame 652.. {
                n139 = Subtract(x=w501, y=w500) -> (x-y=w499:dbl[])
              }
            }
            n140 = call "Savitzky Golay Filter PtByPt with Derivative861.vi"("order polynomial"=w484, "side points"=w485, "x"=w482) -> ("Filtered Derivative"=w476:dbl[], "Filtered x"=w477:dbl[])  [unwired: 1 in, 6 out]
            n141 = Multiply(x=w490, y=w477) -> (x*y=w480:dbl[])
            n142 = Multiply(x=w476, y=w489) -> (x*y=w478:dbl[])
            n143 = Subtract(x=w480, y=w478) -> (x-y=w479:dbl[])
            n144 = Multiply(x=w479, y=w491) -> (x*y=w481:dbl[])
          }
        }
        "last U sample" <- w163
        n145 = case shown="False" "skip feedback" {
          tunnel: w178 -> [_ w208]
          tunnel: w177 -> [_ w207]
          tunnel: w172 -> [_ w206]
          tunnel: w171 -> [_ w205]
          tunnel: [w183 w199] -> w170
          tunnel: [w184 w198] -> w169
          tunnel: w163 -> [_ w195]
          tunnel: w156 -> [_ w194]
          tunnel: w153 -> [_ w193]
          frame True {
            n146 = local read "empty sample array"() -> (w183:dbl[])
            n147 = local read "empty sample array"() -> (w184:dbl[])
          }
          frame False {
            # "it"
            n148 = local read "empty sample array"() -> (w202:dbl[])
            n149 = local read "single channel number"() -> (w204:i64)
            n150 = local read "No. Of Samples to average"() -> (w191:i32)
            n151 = case shown="True" "Use Voltage or Power for AO?" {
              tunnel: w204 -> [w307 w312]
              tunnel: [w308 w311] -> w201
              tunnel: w195 -> [_ w310]
              tunnel: w194 -> [w309 _]
              frame False {
                n152 = Index Array(array=w309, index=w307) -> (element=w308:dbl)
              }
              frame True {
                n153 = Index Array(array=w310, index=w312) -> (element=w311:dbl)
              }
            }
            "single channel voltage" <- w201
            n154 = Quotient & Remainder(x=w193, y=w191) -> (floor(x/y)=→"new level of override":u32)  [unwired: 1 out]
            n155 = local read "voltage factor"() -> (w203:dbl)
            n156 = Multiply(x=w201, y=w203) -> (x*y=w200:dbl)
            n157 = Absolute Value(x=w200) -> (abs(x)=w196:dbl)
            "single channel voltage * factor" <- w196
            n158 = local read "No. Of Samples to average"() -> (w185:i32)
            n159 = Add(x=1, y=w193) -> (x+y=w188:u32)
            n160 = Add(x=w185, y=i64 1) -> (x+y=w186:i64)
            n161 = Replace Array Subset(array=w202, new element=w196, index=w193) -> (w198:dbl[])
            n162 = Greater Or Equal?(x=w188, y=w186) -> (x >= y?=w190:bool)
            "index status" <- w190
            n163 = property class="Arr (strict)"(reference=w208, "Value"=w198) -> ()  [unwired: 1 in, 2 out]
            n164 = case shown="True" w190 {
              tunnel: w193 -> [w209 w227]
              tunnel: w206 -> [w212 w229]
              tunnel: w205 -> [_ w230]
              tunnel: w194 -> [w210 w228]
              tunnel: w185 -> [_ w226]
              tunnel: [_ w225] -> w199
              frame False {
                # "it"
                # "for amount of subselection channels"
                # "no output yet"
                n165 = property class="DigNum (strict)"(reference=w212, "Value"=0.0) -> ()  [unwired: 1 in, 2 out]
                n166 = local read "channelNumber"() -> (w213:i32)
                n167 = for {
                  N: w213 -> [_]
                  tunnel: w209 -> [w220]
                  tunnel: w210 -> [w218]
                  i -> [w215]
                  # "channel"
                  # "channel"
                  # "it+1"
                  n168 = local read "rt prad average array"() -> (w219:dbl[][])
                  n169 = local read "channelSelection"() -> (w224:i64[][])
                  n170 = Index Array(array=w224, index (row)=w215, index (col)=0 ("disabled index (col)")) -> (element=w214:i64)
                  n171 = Add(x=w220, y=1) -> (x+y=w221:u32)
                  n172 = Index Array(array=w218, index=w214) -> (element=w217:dbl)
                  n173 = Replace Array Subset(array=w219, new element=w217, index (row)=w215, index (col)=w221) -> (w216:dbl[][])
                  "rt prad average array" <- w216
                  n174 = local write "rt prad average array"(w216) -> ()
                }
              }
              frame True {
                # "new it"
                # "it % samples2av"
                # "for amount of subselection channels"
                n175 = local read "new level of override"() -> (w240:i32)
                n176 = Multiply(x=w240, y=w226) -> (x*y=w239:i32)
                n177 = Subtract(x=w227, y=w239) -> (x-y=w237:u32)
                n178 = local read "kbolott_and_volume"() -> (w238:dbl[][])
                n179 = local read "channelNumber"() -> (w232:i32)
                n180 = local read "V_cam"() -> (w234:dbl)
                n181 = disable-structure shown="Enabled" {
                  disable-tunnel: [52381772.0 45000000.0] -> w236
                  frame Disabled {
                    # "V_Ptor"
                  }
                  frame Enabled {
                  }
                }
                n182 = for {
                  N: w232 -> [_]
                  tunnel: w238 -> [w275]
                  tunnel: [w280] -> w233
                  tunnel: w228 -> [w280]
                  tunnel: [w260] -> w231
                  tunnel: w237 -> [w260]
                  tunnel: w236 -> [w254]
                  tunnel: 0.53 -> [w258]
                  tunnel: w234 -> [w255]
                  tunnel: w232 -> [w261]
                  tunnel: w227 -> [w266]
                  tunnel: w230 -> [w265]
                  tunnel: w229 -> [w262]
                  tunnel: [w246] -> w225
                  i -> [w259]
                  # "channel number"
                  # "channel number"
                  # "point in av array"
                  # "sample"
                  # "channel number"
                  # "K_bolo"
                  # "Volume"
                  # "channel index"
                  n183 = local read "channelSelection"() -> (w279:i64[][])
                  n184 = Index Array(array=w279, index (row)=w259, index (col)=0 ("disabled index (col)")) -> (element=w276:i64)
                  n185 = local read "No. Of Samples to average"() -> (w248:i32)
                  n186 = Index Array(array=w275, index (row)=w276, index (col)=0 ("disabled index (col)")) -> (element=w256:dbl)
                  n187 = Index Array(array=w275, index (row)=w276, index (col)=1 ("disabled index (col)")) -> (element=w257:dbl)
                  n188 = local read "rt prad average array"() -> (w270:dbl[][])
                  n189 = Array Subset(array=w270, index (row)=w259, length (row)=1, index (col)=1 ("index"), length (col)=w248) -> (w271:dbl[][])
                  n190 = To Double Precision Float(number=w248) -> (double precision float=w247:dbl)
                  n191 = Add Array Elements(numeric array=w271) -> (sum=w244:dbl)
                  n192 = Divide(x=w244, y=w247) -> (x/y=w252:dbl)
                  n193 = Divide(x=w252, y=w258) -> (x/y=w251:dbl)
                  n194 = Multiply(x=w251, y=w257) -> (x*y=w245:dbl)
                  n195 = Divide(x=w245, y=w256) -> (x/y=w250:dbl)
                  n196 = Divide(x=w250, y=w255) -> (x/y=w249:dbl)
                  n197 = Multiply(x=w249, y=w254) -> (x*y=w253:dbl)
                  n198 = Replace Array Subset(array=w270, new element=w253, index (row)=w259, index (col)=0 ("disabled index (col)")) -> (w268:dbl[][])
                  n199 = local write "rt prad average array"(w268) -> ()
                  n200 = Subtract(x=w261, y=i64 1) -> (x-y=w264:i64)
                  n201 = Equal?(x=w264, y=w259) -> (x = y?=w267:bool)
                  n202 = case shown="True" w267 {
                    tunnel: w266 -> [_ w292]
                    tunnel: w265 -> [_ w291]
                    tunnel: w262 -> [_ w290]
                    tunnel: [w281 w284] -> w246
                    frame False {
                      n203 = local read "prad av array"() -> (w281:dbl[])
                    }
                    frame True {
                      w287 = 0 ("index")
                      n204 = local read "channelNumber"() -> (w288:i32)
                      n205 = local read "rt prad average array"() -> (w293:dbl[][])
                      n206 = Array Subset(array=w293, index (row)=w287, length (row)=w288, index (col)=w287, length (col)=1 ("index")) -> (w295:dbl[][])
                      n207 = Add Array Elements(numeric array=w295) -> (sum=w283:dbl)
                      n208 = Divide(x=w283, y=1000000.0) -> (x/y=w285:dbl)
                      n209 = Absolute Value(x=w285) -> (abs(x)=w282:dbl)
                      n210 = local read "prad av array"() -> (w286:dbl[])
                      n211 = property class="DigNum (strict)"(reference=w290, "Value"=w282) -> ()  [unwired: 1 in, 2 out]
                      n212 = Replace Array Subset(array=w286, new element=w282, index=w292) -> (w284:dbl[])
                      n213 = property class="Arr (strict)"(reference=w291, "Value"=w284) -> ()  [unwired: 1 in, 2 out]
                      n214 = local write "prad av array"(w284) -> ()
                    }
                  }
                }
                n215 = local read "channelNumber"() -> (w241:i32)
                n216 = for {
                  N: w241 -> [_]
                  tunnel: w231 -> [w302]
                  tunnel: w233 -> [w300]
                  i -> [w298]
                  # "channel"
                  # "channel"
                  n217 = local read "channelSelection"() -> (w306:i64[][])
                  n218 = Index Array(array=w306, index (row)=w298, index (col)=0 ("disabled index (col)")) -> (element=w296:i64)
                  n219 = Add(x=w302, y=1) -> (x+y=w303:u32)
                  n220 = local read "rt prad average array"() -> (w301:dbl[][])
                  n221 = Index Array(array=w300, index=w296) -> (element=w297:dbl)
                  n222 = Replace Array Subset(array=w301, new element=w297, index (row)=w298, index (col)=w303) -> (w299:dbl[][])
                  n223 = local write "rt prad average array"(w299) -> ()
                }
              }
            }
            n224 = local write "empty sample array"(w198) -> ()
            n225 = property class="DigNum (strict)"(reference=w207, "Value"=w196) -> ()  [unwired: 1 in, 2 out]
          }
        }
        n226 = Replace Array Subset(array=w175, new element=w156, index (col)=w153) -> (w176:sgl[][])  [unwired: 1 in]
        n227 = Replace Array Subset(array=w174, new element=w165, index (col)=w153) -> (w173:sgl[][])  [unwired: 1 in]
        n228 = Replace Array Subset(array=w168, new element=w163, index (col)=w153) -> (w167:sgl[][])  [unwired: 1 in]
      }
    }
  }
  "RawArray" <- w25
  "PowerArray" <- w57
  "real time P_rad array" <- w32
  "single channel voltage array" <- w31
  "AdjustedArray" <- w26
  n229 = call "hComRegStop2013.vi"("error in"=w61, "FPGA VI Reference In"=w62) -> ("error out"=→"error out":errorcluster, "FPGA VI Reference Out"=→"FPGA VI Reference Out":refnum<k20>)  [unwired: 3 in, 1 out]
